vi "Get Configured Audio Device Info.vi"(8 "error in (no error)":errorcluster, 11 "Audio Device Refnum In":T3) -> (0 "error out":errorcluster, 2 "Audio Device Config":T1, 3 "Audio Device Refnum Out":T3)   [LabVIEW 2020, in "G-Audio.lvlib"]
doc: "Get information about the configured audio device."
uses:
  G-Audio.lvlib
  Controls/Audio Device Refnum.ctl
  Controls/Audio Device Config.ctl
  Controls/Audio Device Format.ctl
  <vilib>/Utility/error.llb/Error Cluster From Error Code.vi
  lib/g_audio_32.dll
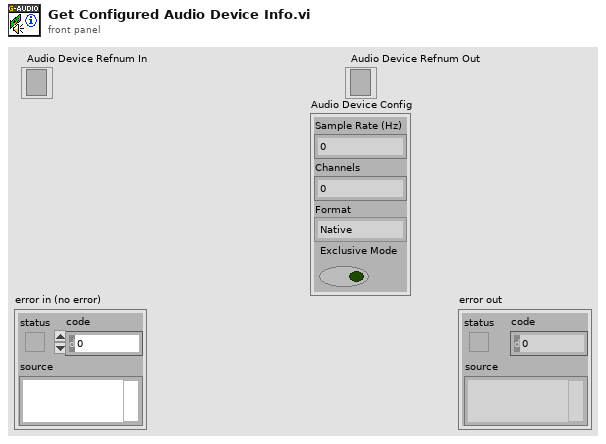
[diagram p1: front panel]
types:
  T1 = typedef "G-Audio.lvlib/Audio Device Config.ctl" = cluster{"Sample Rate (Hz)":u32, "Channels":u32, "Format":T2, "Exclusive Mode":bool}
  T2 = typedef "G-Audio.lvlib/Audio Device Format.ctl" = enum16{"Native", "U8", "I16", "I32", "SGL"}
  T3 = typedef "G-Audio.lvlib/Audio Device Refnum.ctl" = refnum<file>
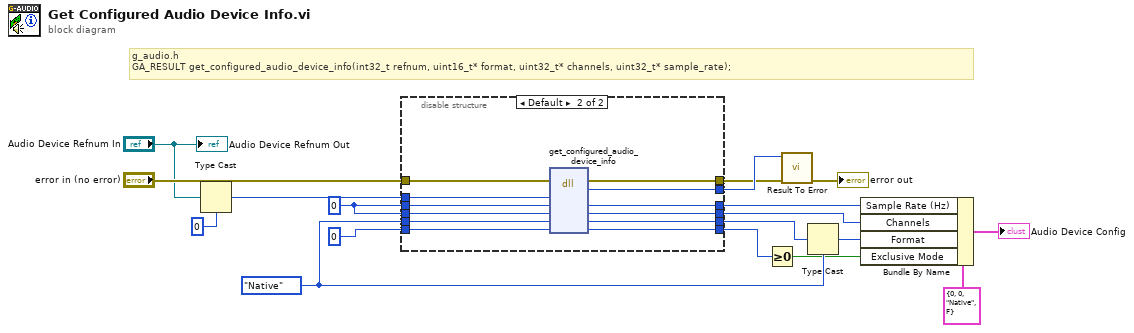
[diagram p0: block diagram]
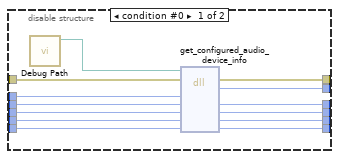
[diagram p2: hidden frame]
diagram:
  w10 = Audio_Device_Format."Native" ("Format")
  w14 = u32 0
  # "g_audio.h\nGA_RESULT get_configured_audio_device_info(int32_t refnum, uint16_t* format, uint32_t* channels, uint32_t* sample_rate);"
  n1 = Type Cast(type=0, x="Audio Device Refnum In") -> (*(type *) &x=w15:i32)
  n2 = disable-structure shown="Default" {
    disable-tunnel: "error in (no error)" -> [w31 w43]
    disable-tunnel: [w28 w40] -> w13
    disable-tunnel: [w30 w42] -> w12
    disable-tunnel: [w23 w36] -> w8
    disable-tunnel: w15 -> [w29 w41]
    disable-tunnel: w14 -> [w25 w38]
    disable-tunnel: w14 -> [w24 w37]
    disable-tunnel: [w22 w35] -> w5
    disable-tunnel: w10 -> [w26 w39]
    disable-tunnel: [w21 w34] -> w6
    disable-tunnel: u8 0 -> [w20 w33]
    disable-tunnel: [w19 w32] -> w3
    frame condition #0 {
      n3 = call "Debug Path.vi"() -> ("Debug Path"=w27:path)  [unwired: 11 in]
      n4 = dll-call lib="?" fn="get_configured_audio_device_info"(path in=w27, error in=w31, "refnum"=w29, "sample_rate"=w25, "channels"=w24, "format"=w26, "exclusive_mode"=w20) -> (error out=w30:errorcluster, "result"=w28:i32, "sample_rate"=w21:u32, "channels"=w22:u32, "format"=w23:u16, "exclusive_mode"=w19:u8)  [unwired: 2 in, 1 out]
    }
    frame condition #1 (active) {
      n5 = dll-call lib="C:/github/dataflowg/g-audio/src/LabVIEW/G-Audio/lib/g_audio_*.*" fn="get_configured_audio_device_info"(error in=w43, "refnum"=w41, "sample_rate"=w38, "channels"=w37, "format"=w39, "exclusive_mode"=w33) -> (error out=w42:errorcluster, "result"=w40:i32, "sample_rate"=w34:u32, "channels"=w35:u32, "format"=w36:u16, "exclusive_mode"=w32:u8)  [unwired: 3 in, 1 out]
    }
  }
  n6 = Greater Or Equal To 0?(x=w3) -> (x >= 0?=w2:bool)
  n7 = call "Result To Error.vi"("error in (no error)"=w12, "Result Code"=w13) -> ("error out"=→"error out":errorcluster)  [unwired: 9 in]
  n8 = Type Cast(type=w10, x=w8) -> (*(type *) &x=w7:T2)
  n9 = Bundle By Name(cluster=T1 {"Sample Rate (Hz)"=0, "Channels"=0, "Format"=enum."Native", "Exclusive Mode"=FALSE} ("Audio Device Config"), "Sample Rate (Hz)"=w6, "Channels"=w5, "Format"=w7, "Exclusive Mode"=w2) -> (→"Audio Device Config":T1)
  "Audio Device Refnum Out" <- "Audio Device Refnum In"
